vi "TestEdgeOn.vi"() -> ()   [LabVIEW 2020]
doc: "Test program for Edge On"
panel:
  out "count":i32
  out "Edge On Found":bool
  in  "Current State":bool
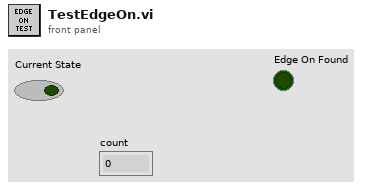
[diagram p1: front panel]
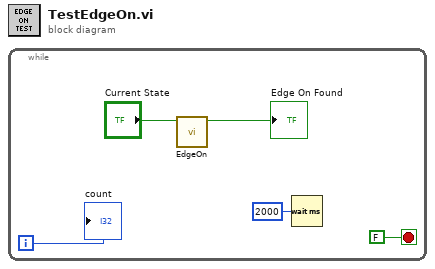
[diagram p0: block diagram]
diagram:
  n1 = while {
    i -> [w1]
    stop <- FALSE stop-if-true
    n2 = call "EdgeOn.vi"("Current State"="Current State") -> ("Edge On Found"=→"Edge On Found":bool)  [unwired: 10 in]
    n3 = Wait (ms)(milliseconds to wait=u32 2000) -> ()  [unwired: 1 out]
    "count" <- w1
  }
